vi "写入数据库(子VI).vi"(7 "数据库选择":u16(ring) items=["使用ACCESS数据库", "使用mySQL数据库"], 8 "error in (no error)":errorcluster, 9 "data":variant, 10 "colums":string[](array[string]), 11 "database":string="database1.mdb") -> (0 "错误输出":errorcluster)   [LabVIEW 2016]
uses:
  <vilib>/Utility/sysdir.llb/System Directory Type.ctl
  <vilib>/addons/database/Connection.llb/DB Tools Open Connec (String).vi
  <vilib>/addons/database/NI_Database_API.lvlib
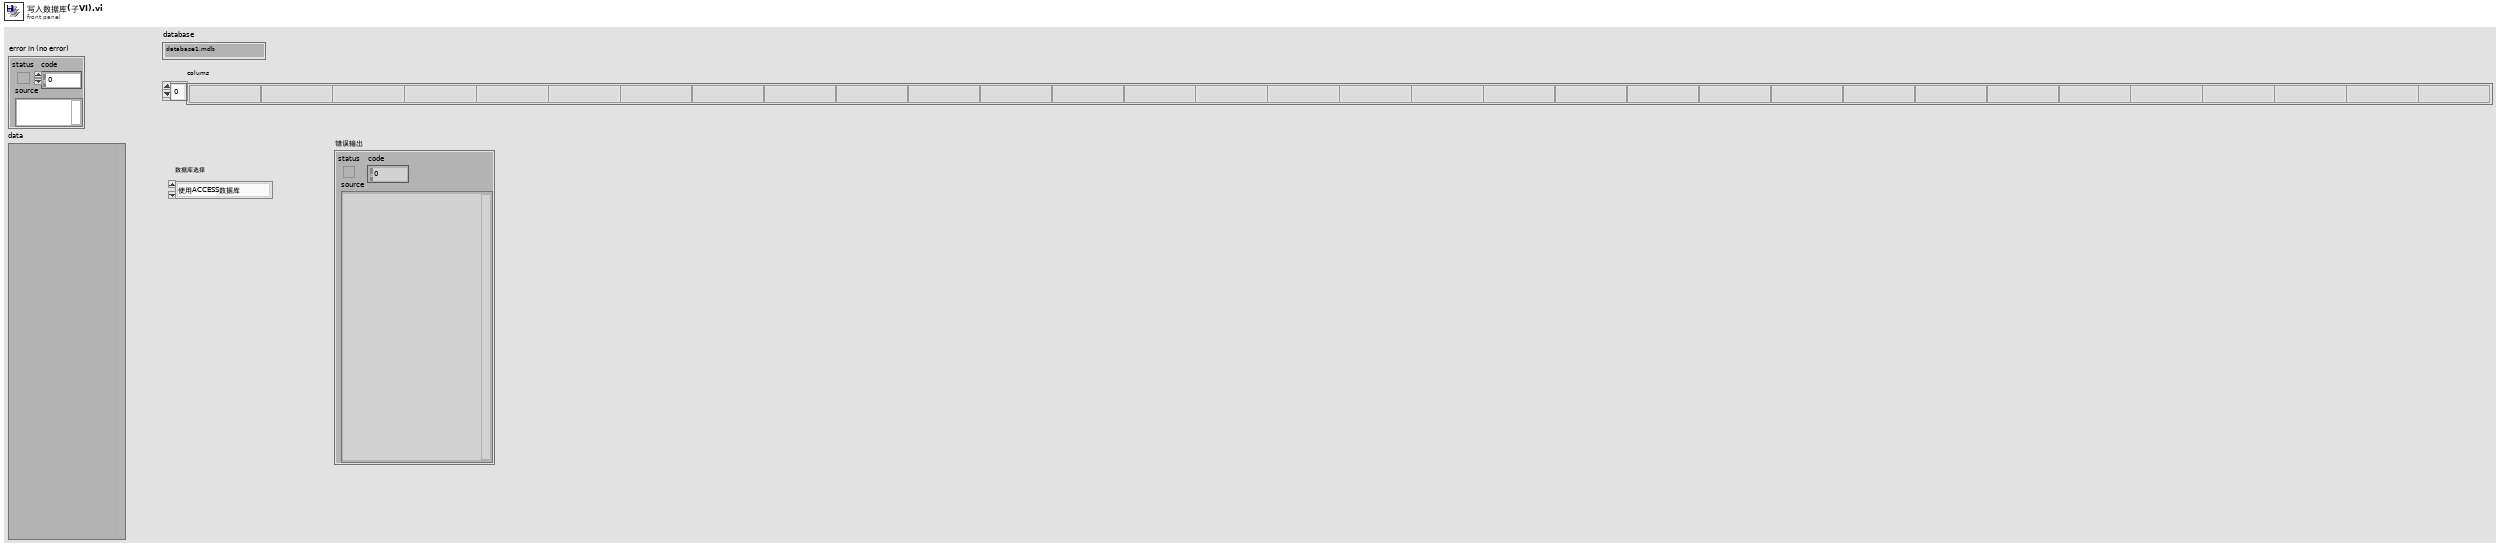
[diagram p1: front panel]
types:
  T1 = typedef "System Directory Type.ctl" = i32
  T2 = typedef "NI_Database_API.lvlib/Conn ObjectReference.ctl" = refnum<k1>
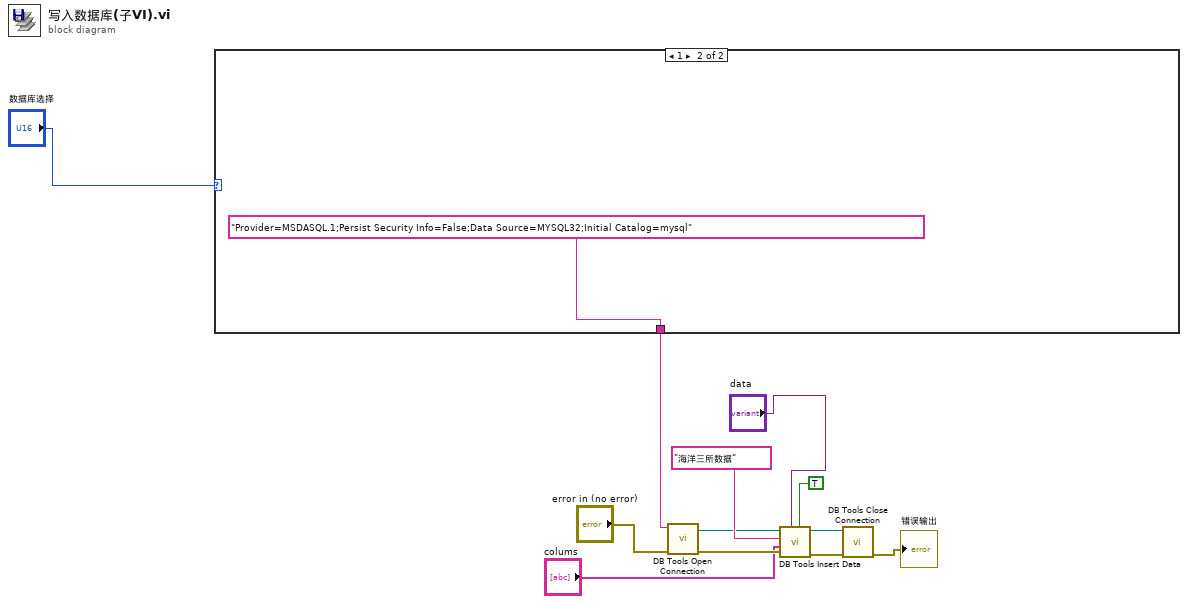
[diagram p0: block diagram]
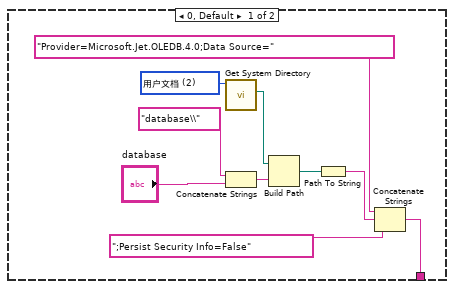
[diagram p2: hidden frame]
diagram:
  n1 = case shown="1" "数据库选择" {
    tunnel: [w22 "Provider=MSDASQL.1;Persist Security Info=False;Data Source=MYSQL32;Initial Catalog=mysql"] -> w5
    frame 0, Default {
      w14 = T1 2 items=["用户目录"=0, "用户桌面"=1, "用户文档"=2, "用户应用程序数据"=3, "用户设置"=4, "用户临时目录"=5, "公共文档"=6, "公共应用程序数据"=7, "公共设置"=8, "公共缓存"=13, "系统核心库"=9, "系统安装库"=10, "应用程序文件"=11, "启动盘根目录"=12] ("system directory type")
      n2 = call <vilib>:"Get System Directory.vi"("system directory type"=w14) -> ("system directory"=w16:path)  [unwired: 10 in]
      n3 = Concatenate Strings("database\\" ("condition"), "database") -> (w20:string)
      n4 = Build Path(base path=w16, name or relative path=w20) -> (appended path=w17:path)
      n5 = Path To String(path=w17) -> (string=w18:string)
      n6 = Concatenate Strings("Provider=Microsoft.Jet.OLEDB.4.0;Data Source=" ("condition"), w18, ";Persist Security Info=False" ("condition")) -> (w22:string)
    }
    frame 1 {
    }
  }
  n7 = call-poly <vilib>:"DB Tools Open Connection.vi"("error in (no error)"="error in (no error)", "connection information"=w5) -> ("error out"=w9:errorcluster, "connection reference"=w6:T2)  [unwired: 6 in]
  n8 = call <vilib>:"DB Tools Insert Data.vi"("create table? (F)"=TRUE, "data"="data", "error in (no error)"=w9, "columns"="colums", "table"="海洋三所数据", "connection reference"=w6) -> ("error out"=w11:errorcluster, "connection reference out"=w10:T2)  [unwired: 4 in]
  n9 = call <vilib>:"DB Tools Close Connection.vi"("error in (no error)"=w11, "connection reference"=w10) -> ("error out"=→"错误输出":errorcluster)  [unwired: 5 in]
